vi "Data.vi"(8 "error in (no error)":errorcluster, 11 "PB Msg Template in":refnum<class "Msg.lvclass">) -> (0 "error out":errorcluster, 2 "Data":T1, 3 "PB Msg Template out":refnum<class "Msg.lvclass">)   [LabVIEW 2020, in "CmdAnalogMultiple.lvlib" / "Msg.lvclass"]
uses:
  Msg.lvclass
  Data.ctl
  CmdAnalog/Data.ctl
  Msg.lvclass/Msg.ctl
  CmdAnalogMultiple.lvlib
  CmdAnalog/CmdAnalog.lvlib
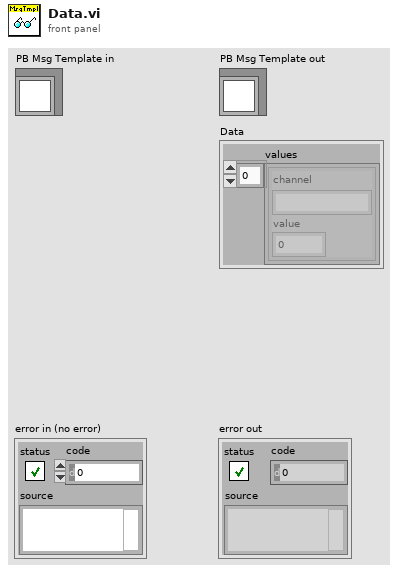
[diagram p1: front panel]
types:
  T1 = typedef "CmdAnalogMultiple.lvlib/Data.ctl" = cluster{"values":T2[]}
  T2 = typedef "CmdAnalog.lvlib/Data.ctl" = cluster{"channel":string, "value":dbl}
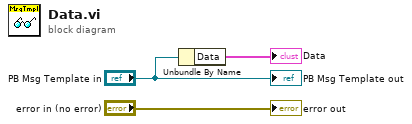
[diagram p0: block diagram]
diagram:
  n1 = Unbundle By Name("PB Msg Template in") -> ("Data"=→"Data":T1)
  "error out" <- "error in (no error)"
  "PB Msg Template out" <- "PB Msg Template in"
